vi "Slack-Dialog (subpanel).vi"(0 "Defaults":path, 5 "client_id":string="1023330033985.1023512746241", 7 "client_secret":string="62f876b60829c507c6cb25bfe9dbba2b", 9 "close event":refnum<user-event>) -> ()   [LabVIEW 2015]
uses:
  Controls/KBackground Gradient/KBackground Gradient.xctl
panel:
  in  "Tab":enum32{"Page 1", "Page 2"}(tab)
  out "Channel":string
  out "Workspace":string
  out "Users":string caption="channel"
  in  "Refresh Button":bool
  in  "Sign in Button":bool
  in  "Gradient":dbl(xcontrol)
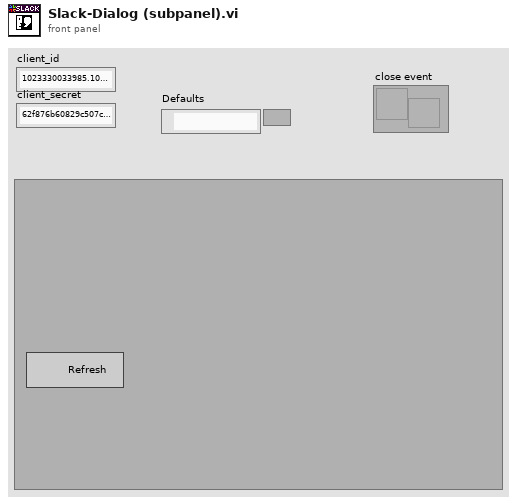
[diagram p1: front panel]
types:
  T1 = typedef "Slack-Configuration.ctl" = cluster{"app_id":string, "authed_user":cluster{"id":string}, "access_token":string, "bot_user_id":string, "team":cluster{"id":string, "name":string}, "bot channel":cluster{"id":string, "name":string}, "bot_user_name":string}
  T2 = typedef "Slack-User.ctl" = cluster{"id":string, "name":string}
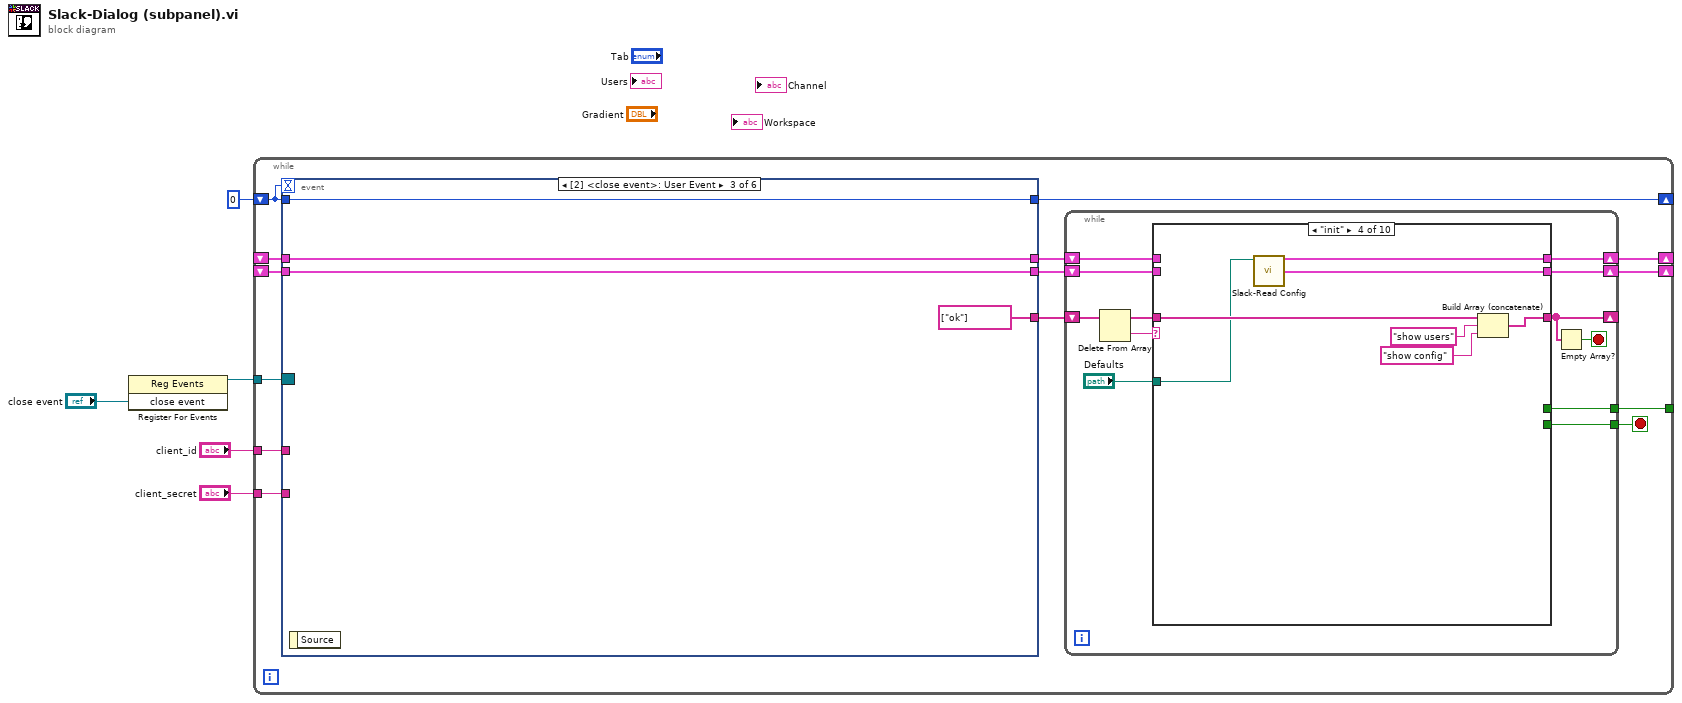
[diagram p0: block diagram]
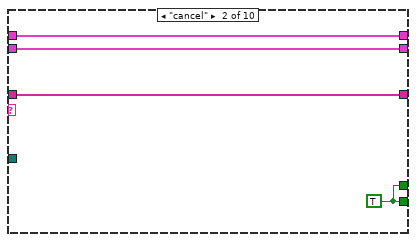
[diagram p3: hidden frame]
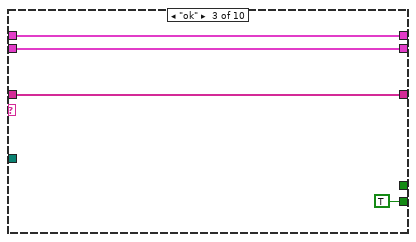
[diagram p4: hidden frame]
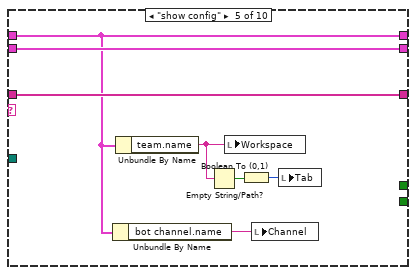
[diagram p5: hidden frame]
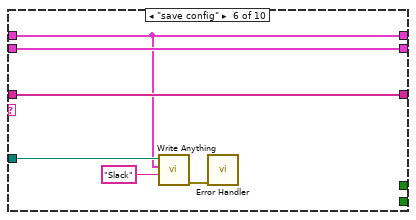
[diagram p6: hidden frame]
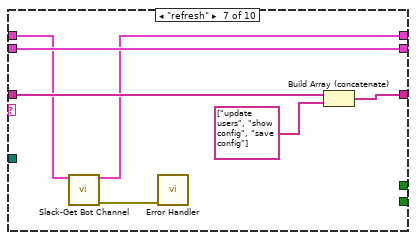
[diagram p7: hidden frame]
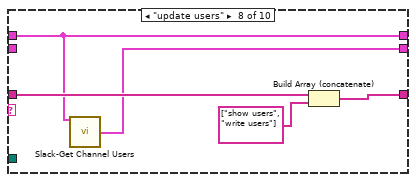
[diagram p8: hidden frame]
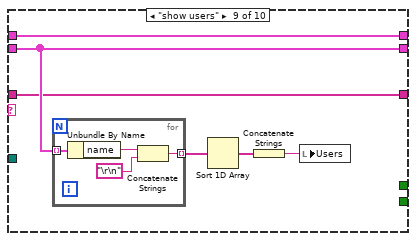
[diagram p9: hidden frame]
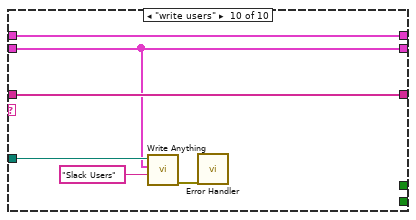
[diagram p10: hidden frame]
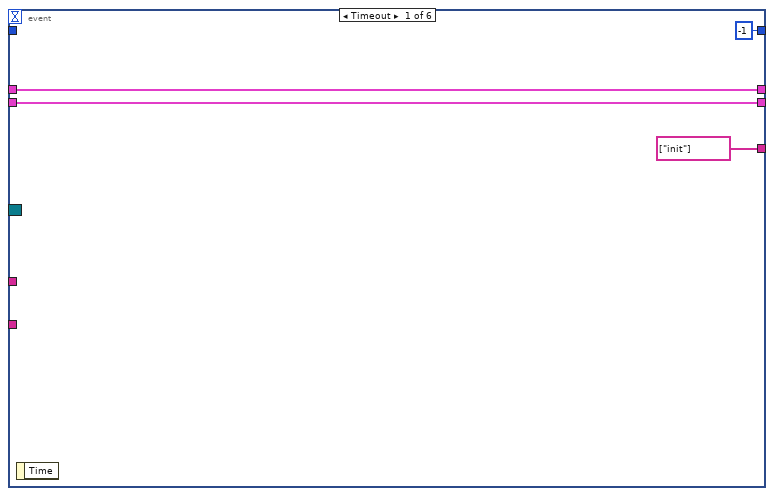
[diagram p11: hidden frame]
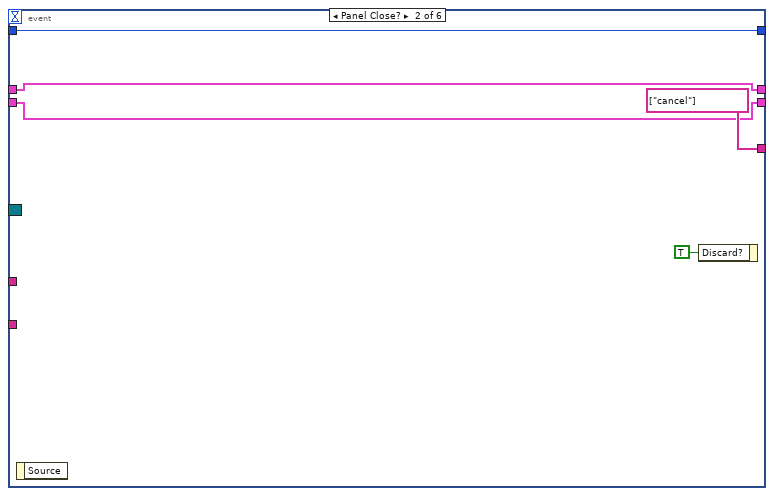
[diagram p12: hidden frame]
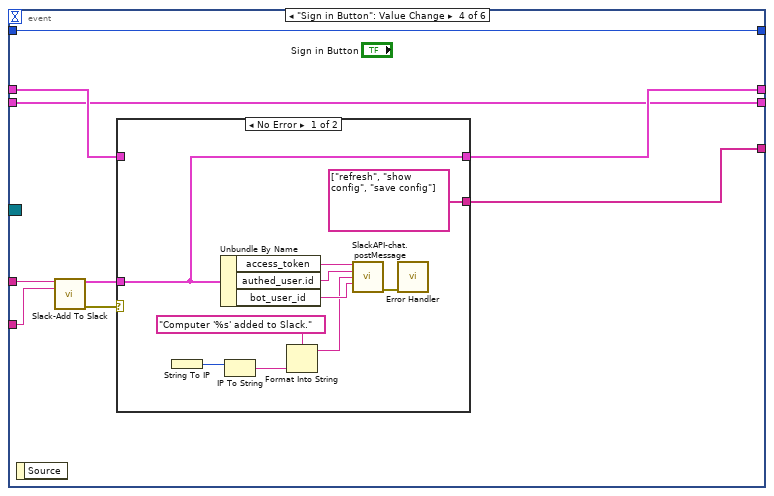
[diagram p13: hidden frame]
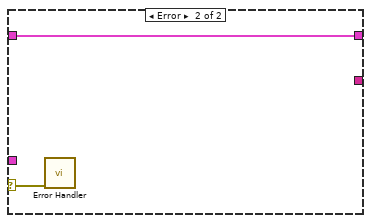
[diagram p14: hidden frame]
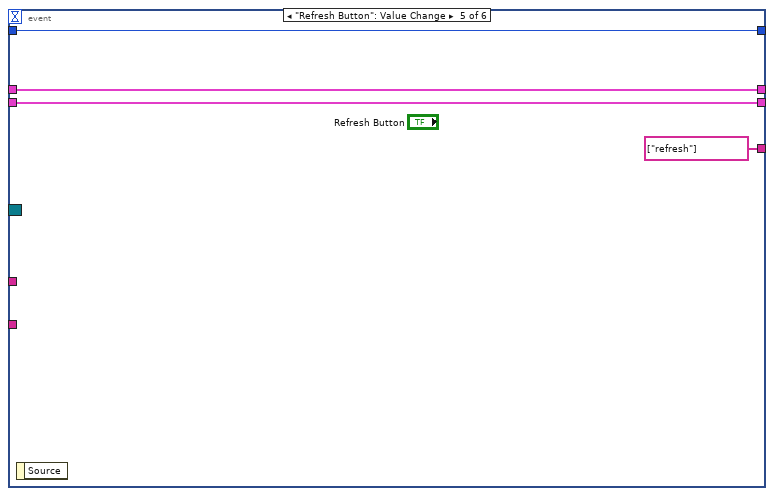
[diagram p15: hidden frame]
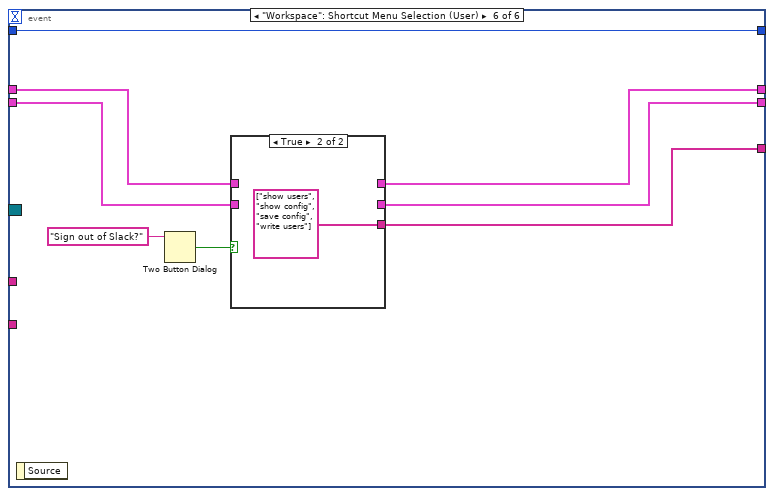
[diagram p16: hidden frame]
diagram:
  n1 = register-events("close event") -> (reference out=w1:refnum<event-registration>)  [unwired: 2 in, 1 out]
  n2 = while {
    shift-right: [w19] -> _
    shift-left: 0 -> [w18]
    tunnel: [w15] -> _
    shift-right: [w14] -> _
    shift-left: _ -> [w12]
    shift-right: [w11] -> _
    shift-left: _ -> [w9]
    tunnel: "client_id" -> [w8]
    tunnel: "client_secret" -> [w7]
    tunnel: w1 -> [w6]
    stop <- w16 stop-if-true
    n3 = event shown="[2] <close event>: User Event" {
      selector: w6 -> [_ _ _ _ _ _]
      dyn-events: _ -> [_ _ _ _ _ _]
      timeout: w18 -> [_ _ _ _ _ _]
      tunnel: [-1 w99 w103 w112 w128 w136] -> w19
      tunnel: w18 -> [_ w99 w103 w112 w128 w136]
      tunnel: [string[] ["init"] string[] ["cancel"] string[] ["ok"] w104 string[] ["refresh"] w129] -> w17
      tunnel: [w92 w96 w101 w108 w127 w132] -> w13
      tunnel: w12 -> [w92 w96 w101 w107 w127 w133]
      tunnel: [w91 w95 w100 w105 w126 w130] -> w10
      tunnel: w9 -> [w91 w95 w100 w105 w126 w131]
      tunnel: w8 -> [_ _ _ w111 _ _]
      tunnel: w7 -> [_ _ _ w110 _ _]
      event Timeout {
        n4 = event-data() -> ()  [unwired: 1 in, 1 out]
      }
      event Panel Close? {
        n5 = event-data() -> ()  [unwired: 1 in, 1 out]
        n6 = event-data("Discard?"=TRUE) -> ()  [unwired: 1 in, 1 out]
      }
      event User Event {
        n7 = event-data() -> ()  [unwired: 1 in, 1 out]
      }
      event "Sign in Button": Value Change {
        n8 = event-data() -> ()  [unwired: 1 in, 1 out]
        n9 = call "Slack-Add To Slack.vi"("client_id"=w111, "client_secret"=w110) -> ("config"=w106:T1, "error out"=w109:errorcluster)  [unwired: 12 in]
        n10 = case shown="No Error" w109 {
          selector: w109 -> [_ w123]
          tunnel: [w118 w124] -> w108
          tunnel: w107 -> [_ w124]
          tunnel: w106 -> [w118 _]
          tunnel: [string[] ["refresh", "show config", "save config"] _] -> w104
          frame No Error {
            n11 = String To IP() -> (0:w121:u32)  [unwired: 1 in]
            n12 = Unbundle By Name(w118) -> ("access_token"=w117:string, "authed_user.id"=w116:string, "bot_user_id"=w115:string)
            n13 = IP To String(2:w121) -> (0:w119:string)  [unwired: 1 in]
            n14 = Format Into String(format string="Computer '%s' added to Slack.", w119) -> (resulting string=w114:string)  [unwired: 2 in, 1 out]
            n15 = call "SlackAPI-chat.postMessage.vi"("access_token"=w117, "user ID"=w116, "message"=w114, "username"=w115) -> ("error out"=w113:errorcluster)  [unwired: 11 in]
            n16 = call "Error Handler.vi"("error in (no error)"=w113) -> ()  [unwired: 13 in, 2 out]
          }
          frame Error {
            n17 = call "Error Handler.vi"("error in (no error)"=w123) -> ()  [unwired: 13 in, 2 out]
          }
        }
      }
      event "Refresh Button": Value Change {
        n18 = event-data() -> ()  [unwired: 1 in, 1 out]
      }
      event "Workspace": Shortcut Menu Selection (User) {
        n19 = event-data() -> ()  [unwired: 1 in, 1 out]
        n20 = Two Button Dialog(message="Sign out of Slack?" ("T button name (\"OK\")")) -> (T button?=w134:bool)  [unwired: 2 in]
        n21 = case shown="True" w134 {
          tunnel: w131 -> [w137 _]
          tunnel: w133 -> [w138 _]
          tunnel: [w138 _] -> w132
          tunnel: [w137 _] -> w130
          tunnel: [_ string[] ["show users", "show config", "save config", "write users"]] -> w129
          frame False {
          }
          frame True {
          }
        }
      }
    }
    n22 = while {
      shift-right: [w20] -> _
      shift-left: w17 -> [w31]
      tunnel: [w27] -> w16
      tunnel: [w26] -> w15
      shift-right: [w25] -> w14
      shift-left: w13 -> [w24]
      shift-right: [w23] -> w11
      shift-left: w10 -> [w22]
      stop <- w28 stop-if-true
      n23 = Delete From Array(array=w31) -> (deleted portion=w29:string, array with subset deleted=w30:string[])  [unwired: 2 in]
      n24 = case shown="\"init\"" w29 {
        tunnel: w30 -> [w32 w35 w39 w49 w56 w62 w69 w74 w77 w90]
        tunnel: [w32 w35 w39 w47 w56 w62 w64 w73 w77 w90] -> w20
        tunnel: [_ w38 TRUE _ _ _ _ _ _ _] -> w27
        tunnel: [_ w38 _ _ _ _ _ _ _ _] -> w26
        tunnel: [w34 w37 w41 w43 w51 w58 w65 w71 w79 w89] -> w25
        tunnel: w24 -> [w34 w37 w41 _ w51 w58 w66 w71 w79 w89]
        tunnel: [w33 w36 w40 w48 w52 w61 w68 w70 w78 w87] -> w23
        tunnel: w22 -> [w33 w36 w40 _ w52 w61 w68 _ w78 w87]
        tunnel: "Defaults" -> [_ _ _ w45 _ w59 _ _ _ w88]
        frame "", Default {
        }
        frame "cancel" {
          w38 = TRUE
        }
        frame "ok" {
        }
        frame "init" {
          n25 = call "Slack-Read Config.vi"("AppName"=w45) -> ("config"=w43:T1, "users"=w48:T2[])  [unwired: 12 in, 1 out]
          n26 = Build Array (concatenate)(w49, "show users", "show config") -> (w47:string[])
        }
        frame "show config" {
          n27 = Unbundle By Name(w51) -> ("bot channel.name"=w50:string)
          n28 = Unbundle By Name(w51) -> ("team.name"=w54:string)
          n29 = Empty String/Path?(string/path=w54) -> (empty?=w53:bool)
          n30 = local write "Workspace"(w54) -> ()
          n31 = Boolean To (0,1)(Boolean=w53) -> (0, 1=w55:i16)
          n32 = local write "Channel"(w50) -> ()
          n33 = local write "Tab"(w55) -> ()
        }
        frame "save config" {
          n34 = call "Write Anything.vi"("Section Name (Name of \"Anything\")"="Slack" ("Section Name (Name of \"Anything\")"), "Anything"=w58, "Path (dialog)"=w59) -> ("Error Out"=w57:errorcluster)  [unwired: 7 in, 1 out]
          n35 = call "Error Handler.vi"("error in (no error)"=w57) -> ()  [unwired: 13 in, 2 out]
        }
        frame "refresh" {
          n36 = call "Slack-Get Bot Channel.vi"("config in"=w66) -> ("config out"=w65:T1, "error out"=w67:errorcluster)  [unwired: 13 in]
          n37 = call "Error Handler.vi"("error in (no error)"=w67) -> ()  [unwired: 13 in, 2 out]
          n38 = Build Array (concatenate)(w69, string[] ["update users", "show config", "save config"]) -> (w64:string[])
        }
        frame "update users" {
          n39 = call "Slack-Get Channel Users.vi"("config in"=w71) -> ("users"=w70:T2[])  [unwired: 13 in, 1 out]
          n40 = Build Array (concatenate)(w74, string[] ["show users", "write users"]) -> (w73:string[])
        }
        frame "show users" {
          n41 = for {
            tunnel: w78 -> [w84] mode=indexing
            tunnel: [w82] -> w80 mode=indexing
            n42 = Unbundle By Name(w84) -> ("name"=w83:string)
            n43 = Concatenate Strings(w83, "\r\n") -> (w82:string)
          }
          n44 = Sort 1D Array(array=w80) -> (sorted array=w76:string[])
          n45 = Concatenate Strings(w76) -> (w75:string)
          n46 = local write "Users"(w75) -> ()
        }
        frame "write users" {
          n47 = call "Write Anything.vi"("Section Name (Name of \"Anything\")"="Slack Users" ("Section Name (Name of \"Anything\")"), "Anything"=w87, "Path (dialog)"=w88) -> ("Error Out"=w85:errorcluster)  [unwired: 7 in, 1 out]
          n48 = call "Error Handler.vi"("error in (no error)"=w85) -> ()  [unwired: 13 in, 2 out]
        }
      }
      n49 = Empty Array?(array=w20) -> (empty?=w28:bool)
    }
  }
